vi "Update Blink.vi"(11 "Blinker in":refnum<class "Blinker.lvclass">) -> (3 "Blinker out":refnum<class "Blinker.lvclass">)   [LabVIEW 2015, in "Blinker.lvclass"]
uses:
  Blinker.lvclass
  Blinker.lvclass/Blinker.ctl
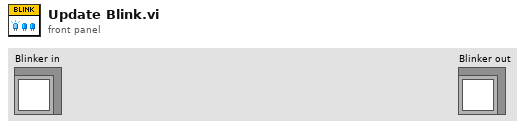
[diagram p1: front panel]
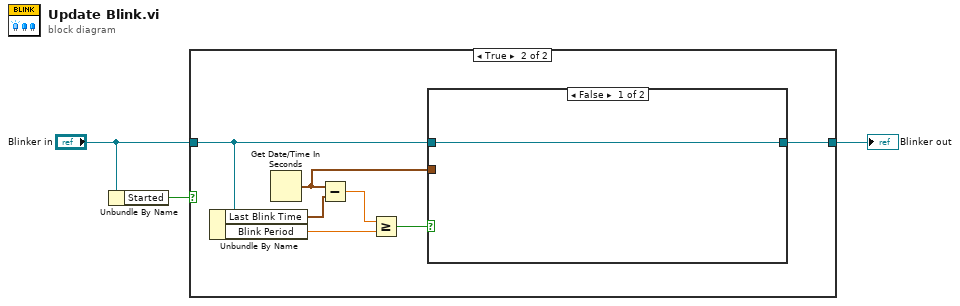
[diagram p0: block diagram]
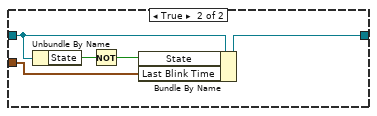
[diagram p3: hidden frame]
diagram:
  n1 = Unbundle By Name("Blinker in") -> ("Started"=w3:bool)
  n2 = case shown="True" w3 {
    tunnel: [w4 w5] -> w2
    tunnel: "Blinker in" -> [w4 w7]
    frame False {
    }
    frame True {
      n3 = Unbundle By Name(w7) -> ("Last Blink Time"=w11:timestamp, "Blink Period"=w9:dbl)
      n4 = Get Date/Time In Seconds() -> (seconds since 1Jan1904=w6:timestamp)
      n5 = Subtract(x=w6, y=w11) -> (x-y=w10:dbl)
      n6 = Greater Or Equal?(x=w10, y=w9) -> (x >= y?=w8:bool)
      n7 = case shown="False" w8 {
        tunnel: w7 -> [w12 w17]
        tunnel: w6 -> [_ w14]
        tunnel: [w12 w13] -> w5
        frame False {
        }
        frame True {
          n8 = Unbundle By Name(w17) -> ("State"=w16:bool)
          n9 = Not(x=w16) -> (.not. x?=w15:bool)
          n10 = Bundle By Name(cluster=w17, "State"=w15, "Last Blink Time"=w14) -> (w13:refnum<class "Blinker.lvclass">)
        }
      }
    }
  }
  "Blinker out" <- w2
